vi "ANDOR_GetHardwareVersion.vi"(7 "error in (no error)":errorcluster) -> (18 "Hardware Versions":cluster{"PCB":u32, "Flex":u32}, 20 "PCB":u32, 21 "Flex":u32, 22 "dummy1":u32, 23 "dummy2":u32, 24 "dummy3":u32, 25 "dummy4":u32, 26 "DLL error code":u32, 27 "error out":errorcluster)   [LabVIEW 2010]
doc: "This function returns the Hardware version information.\n\n<B>Parameters:</B>\nPCB - Plug-in card version\nFlex - Flex 10K file version\n\n<B>Error codes:</B>\nDRV_SUCCESS - Version information returned.\nDRV_NOT_INITIALIZED - System not initialized.\nDRV_ACQUIRING - Acquisition in progress.\nDRV_ERROR_ACK - Unable to communicate with card."
uses:
  Program Files/Andor SOLIS/atmcd32d.dll
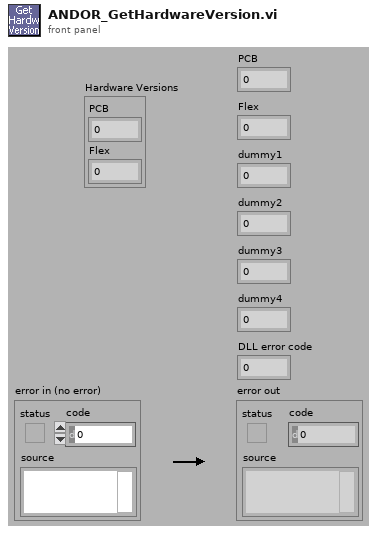
[diagram p1: front panel]
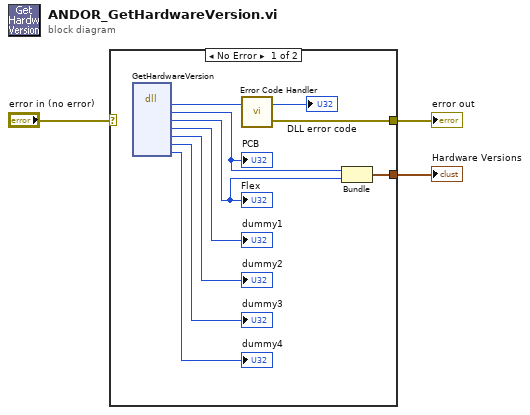
[diagram p0: block diagram]
diagram:
  n1 = case shown="No Error" "error in (no error)" {
    selector: "error in (no error)" -> [_ w14]
    tunnel: [w12 w14] -> w2
    tunnel: [w4 _] -> w1
    frame No Error {
      n2 = dll-call lib="C:/Program Files/Andor SOLIS/atmcd32d.dll" fn="GetHardwareVersion"() -> ("return type"=w13:u32, "PCB"=w6:u32, "Flex"=w5:u32, "dummy1"=→"dummy1":u32, "dummy2"=→"dummy2":u32, "dummy3"=→"dummy3":u32, "dummy4"=→"dummy4":u32)  [unwired: 9 in, 2 out]
      "PCB" <- w6
      "Flex" <- w5
      n3 = call <userlib>:"Error Code Handler.vi"("DLL error code"=w13) -> ("error out"=w12:errorcluster, "dup DLL error code"=→"DLL error code":u32)  [unwired: 1 in]
      n4 = Bundle("PCB"=w6, "Flex"=w5) -> (w4:cluster{"PCB":u32, "Flex":u32})  [unwired: 1 in]
    }
    frame Error {
    }
  }
  "error out" <- w2
  "Hardware Versions" <- w1
